vi "DriveAuto.vi"(8 "DriveAutoInput":T3, 11 "GeneralAutoInput":T2) -> (3 "AutoGeneralOut":T1)   [LabVIEW 2017]
uses:
  AutoSubsystem/AutoOutput.ctl
  AutoSubsystem/AutoSubroutine.lvclass
  AutoSubsystem/AutoDrive/AutoDrive.lvclass
  DriveAutoData.ctl
  AutoSubsystem/AutoInput.ctl
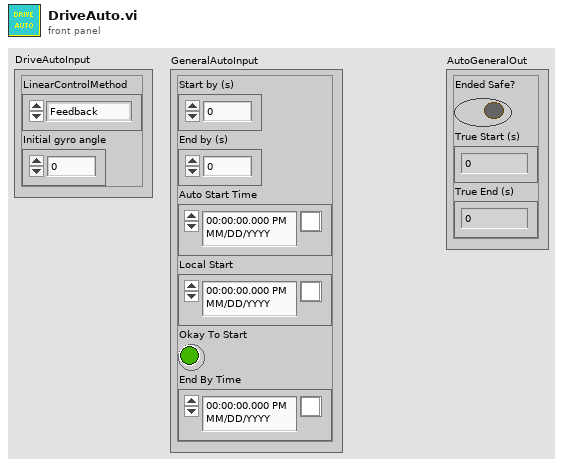
[diagram p1: front panel]
types:
  T1 = typedef "AutoSubroutine.lvclass/AutoOutput.ctl" = cluster{"Ended Safe?":bool, "True Start (s)":dbl, "True End (s)":dbl}
  T2 = typedef "AutoSubroutine.lvclass/AutoInput.ctl" = cluster{"Start by (s)":dbl, "End by (s)":dbl, "Auto Start Time":timestamp, "Local Start":timestamp, "Okay To Start":bool, "End By Time":timestamp}
  T3 = typedef "AutoDrive.lvclass/DriveAutoData.ctl" = cluster{"LinearControlMethod":enum16{"Feedback", "Time"}, "Initial gyro angle":dbl}
  T4 = typedef "AutoDrive.lvclass/DriveAutoDirections.ctl" = cluster{"Forward/Reverse":enum16{"Forward", "Reverse"}, "Right/Left":enum16{"Right/CW", "Left/CCW"}}
  T5 = cluster{"Arc Difference":dbl, "Angle":dbl, "Linear Value":dbl}
  T6 = typedef "DriveMode.lvclass/DriveAutoType.ctl" = enum16{"Straight", "Spin", "Arc"}
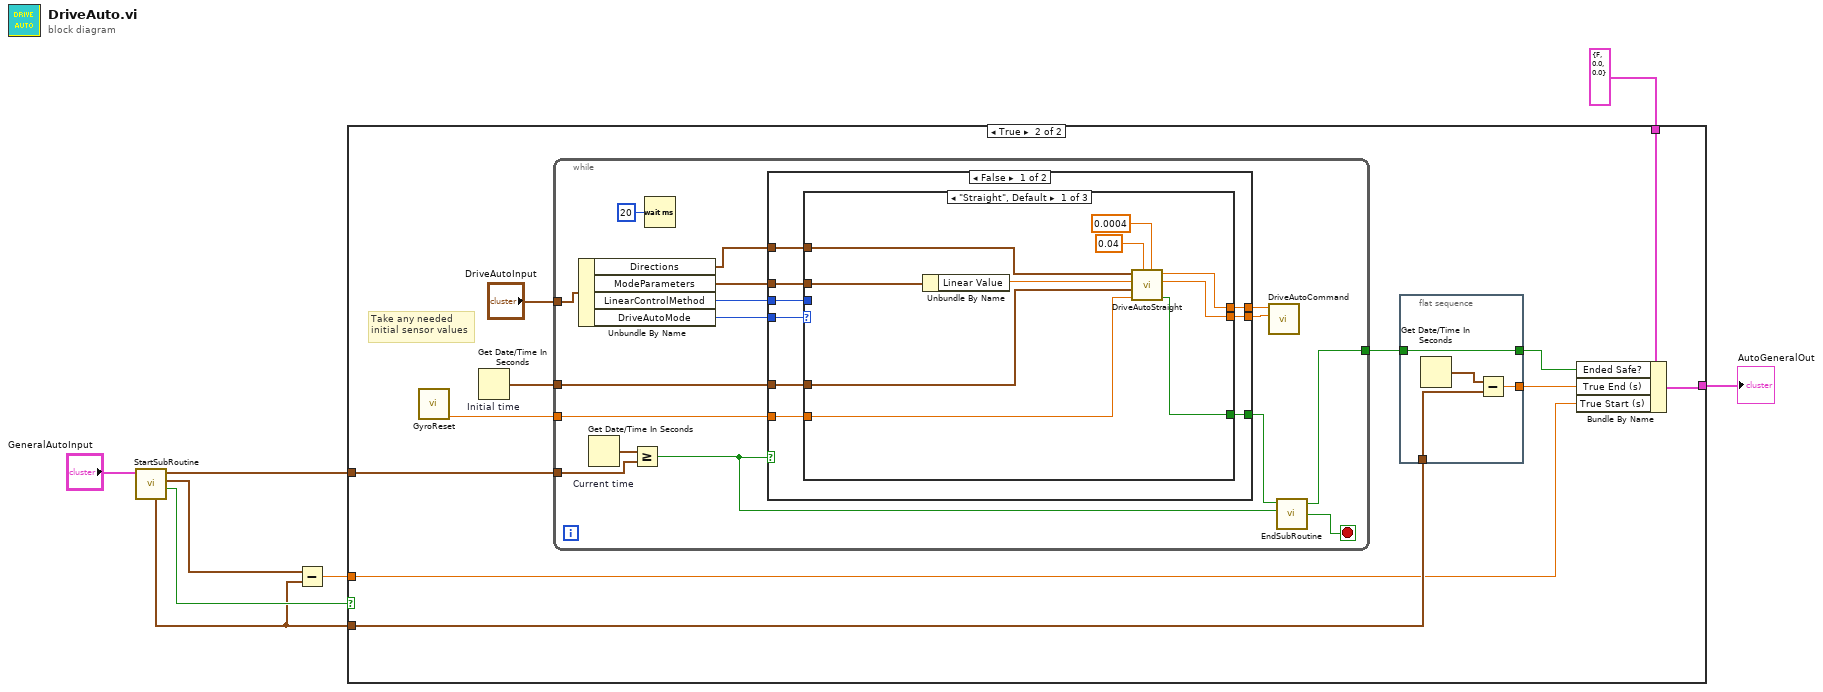
[diagram p0: block diagram]
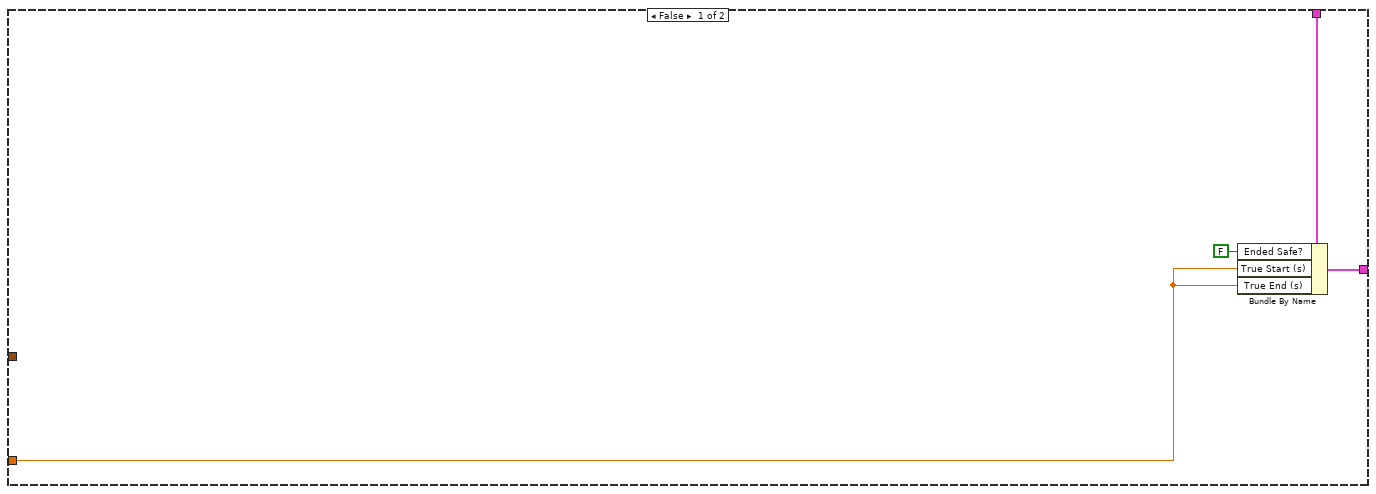
[diagram p2: hidden frame]
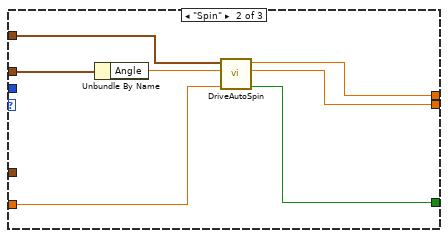
[diagram p3: hidden frame]
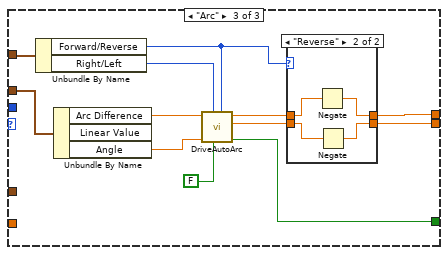
[diagram p4: hidden frame]
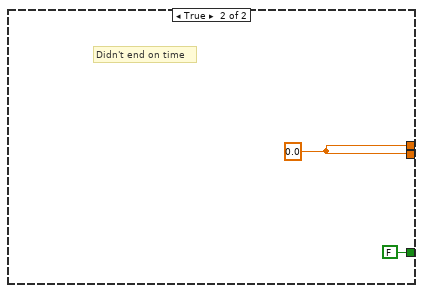
[diagram p6: hidden frame]
diagram:
  n1 = call "StartSubRoutine.vi"("GeneralAutoInput"="GeneralAutoInput") -> ("Okay to start?"=w4:bool, "Local Start"=w3:timestamp, "End by:"=w5:timestamp, "Auto Start Time"=w2:timestamp)  [unwired: 7 in]
  n2 = Subtract(x=w3, y=w2) -> (x-y=w1:dbl)
  n3 = case shown="True" w4 {
    tunnel: [w11 w20] -> w8
    tunnel: w5 -> [_ w22]
    tunnel: T1 {"Ended Safe?"=FALSE, "True Start (s)"=0.0, "True End (s)"=0.0} ("AutoGeneralOut 2") -> [w12 w21]
    tunnel: w2 -> [_ w19]
    tunnel: w1 -> [w9 w18]
    frame False {
      n4 = Bundle By Name(cluster=w12, "Ended Safe?"=FALSE, "True Start (s)"=w9, "True End (s)"=w9) -> (w11:T1)
    }
    frame True {
      # "Take any needed\ninitial sensor values"
      n5 = call "GyroReset.vi"() -> ("Heading"=w13:dbl)  [unwired: 11 in]
      n6 = Get Date/Time In Seconds "Initial time"() -> (seconds since 1Jan1904=w14:timestamp)
      n7 = while {
        tunnel: "DriveAutoInput" -> [w39]
        tunnel: w22 -> [w42]
        tunnel: [w34] -> w15
        tunnel: w13 -> [w33]
        tunnel: w14 -> [w31]
        stop <- w35 stop-if-true
        n8 = Unbundle By Name(w39) -> ("Directions"=w37:T4, "ModeParameters"=w38:T5, "LinearControlMethod"=w40:enum16{"Feedback", "Time"}, "DriveAutoMode"=w41:T6)
        n9 = Get Date/Time In Seconds "Current time"() -> (seconds since 1Jan1904=w43:timestamp)
        n10 = Greater Or Equal?(x=w43, y=w42) -> (x >= y?=w30:bool)
        n11 = Wait (ms)(milliseconds to wait=u32 20) -> ()  [unwired: 1 out]
        n12 = case shown="False" w30 {
          tunnel: w41 -> [w52 _]
          tunnel: w40 -> [w51 _]
          tunnel: w38 -> [w50 _]
          tunnel: w37 -> [w49 _]
          tunnel: [w48 FALSE ("Done?")] -> w36
          tunnel: w33 -> [w47 _]
          tunnel: w31 -> [w46 _]
          tunnel: [w45 w88] -> w29
          tunnel: [w44 w88] -> w28
          frame False {
            n13 = case shown="\"Straight\", Default" w52 {
              tunnel: w51 -> [_ _ _]
              tunnel: w50 -> [w62 w69 w81]
              tunnel: w49 -> [w61 w65 w80]
              tunnel: [w57 w68 w74] -> w48
              tunnel: w47 -> [w60 w67 _]
              tunnel: w46 -> [w53 _ _]
              tunnel: [w54 w63 w71] -> w45
              tunnel: [w55 w64 w70] -> w44
              frame "Straight", Default {
                n14 = Unbundle By Name(w62) -> ("Linear Value"=w56:dbl)
                n15 = call "DriveAutoStraight.vi"("D Gain"=0.0004, "P Gain"=0.04, "Initial Angle"=w60, "Initial Time"=w53, "Target Distance (feet)"=w56, "Directions"=w61) -> ("Done?"=w57:bool, "Right Motor Value"=w54:dbl, "Left Motor Value"=w55:dbl)  [unwired: 3 in]
              }
              frame "Spin" {
                n16 = Unbundle By Name(w69) -> ("Angle"=w66:dbl)
                n17 = call "DriveAutoSpin.vi"("Current Heading"=w67, "Target Angle"=w66, "Directions"=w65) -> ("Done?"=w68:bool, "Right Motor Value"=w63:dbl, "Left Motor Value"=w64:dbl)  [unwired: 6 in]
              }
              frame "Arc" {
                n18 = Unbundle By Name(w80) -> ("Forward/Reverse"=w73:enum16{"Forward", "Reverse"}, "Right/Left"=w75:enum16{"Right/CW", "Left/CCW"})
                n19 = Unbundle By Name(w81) -> ("Arc Difference"=w76:dbl, "Angle"=w77:dbl)  [unwired: 1 out]
                n20 = call "DriveAutoArc.vi"("Forward/Reverse"=w73, "Use Distance?"=FALSE, "Right/Left"=w75, "End value (dist or angle)"=w77, "Arc Difference"=w76) -> ("Done?"=w74:bool, "Right Drive Value"=w78:dbl, "Left Drive Value"=w79:dbl)  [unwired: 4 in]
                n21 = case shown="\"Reverse\"" w73 {
                  tunnel: w79 -> [w83 w87]
                  tunnel: w78 -> [w82 w86]
                  tunnel: [w82 w85] -> w71
                  tunnel: [w83 w84] -> w70
                  frame "Forward", Default {
                  }
                  frame "Reverse" {
                    n22 = Negate(x=w87) -> (-x=w84:dbl)
                    n23 = Negate(x=w86) -> (-x=w85:dbl)
                  }
                }
              }
            }
          }
          frame True {
            w88 = 0.0
            # "Didn't end on time"
          }
        }
        n24 = call "DriveAutoCommand.vi"("RightDriveMagnatude"=w29, "LeftDriveMagnatude"=w28) -> ()  [unwired: 10 in]
        n25 = call "EndSubRoutine.vi"("Done?"=w36, "Ran too long?"=w30) -> ("Safe Stop?"=w34:bool, "Stop?"=w35:bool)  [unwired: 5 in]
      }
      n26 = flat-sequence {
        tunnel: w19 -> [w26]
        tunnel: [w25] -> w17
        tunnel: [w24] -> w16
        tunnel: w15 -> [w24]
        frame #0 {
          n27 = Get Date/Time In Seconds() -> (seconds since 1Jan1904=w27:timestamp)
          n28 = Subtract(x=w27, y=w26) -> (x-y=w25:dbl)
        }
      }
      n29 = Bundle By Name(cluster=w21, "Ended Safe?"=w16, "True End (s)"=w17, "True Start (s)"=w18) -> (w20:T1)
    }
  }
  "AutoGeneralOut" <- w8
